vi "findMark&&ServiceItems.vi"(0 "priceListData":string[][](array[string]), 7 "Numeric":i32, 11 "error in (no error)":errorcluster) -> (8 "found?":bool, 15 "error IO":errorcluster)   [LabVIEW 2012]
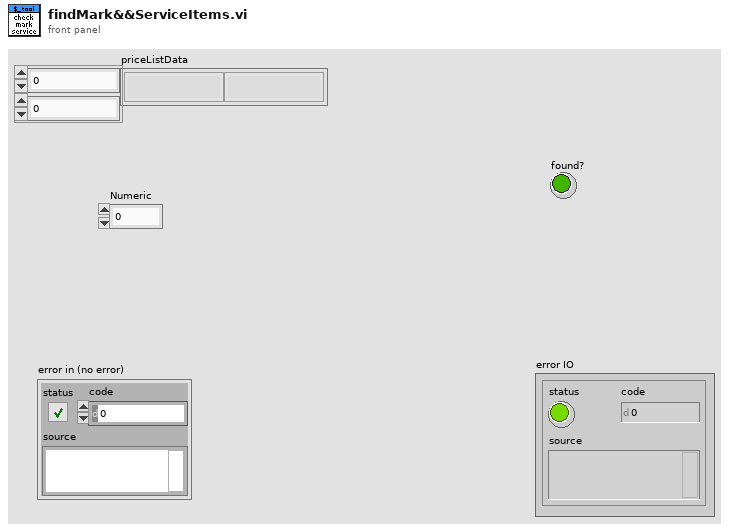
[diagram p1: front panel]
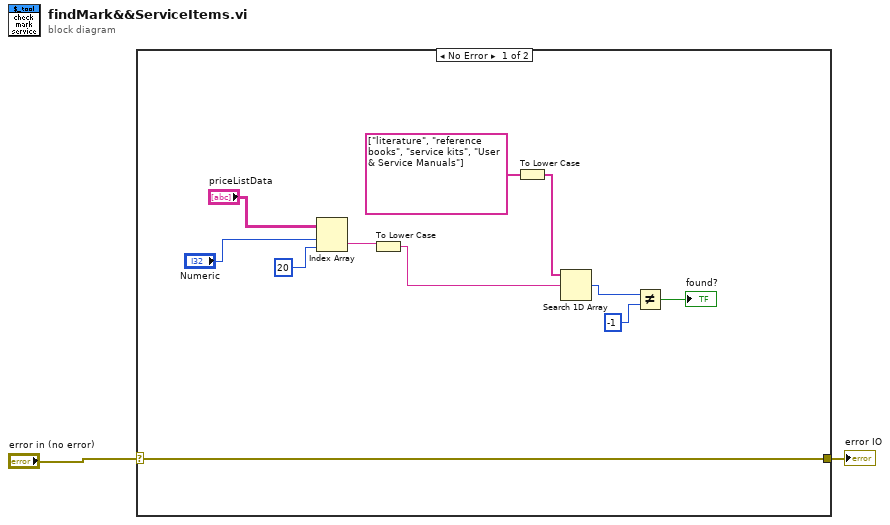
[diagram p0: block diagram]
diagram:
  n1 = case shown="No Error" "error in (no error)" {
    selector: "error in (no error)" -> [w13 w14]
    tunnel: [w13 w14] -> w1
    frame No Error {
      n2 = Index Array(array="priceListData", index (row)="Numeric", index (col)=20 ("disabled index (col)")) -> (element=w9:string)
      n3 = To Lower Case(string=w9) -> (all lower case string=w8:string)
      n4 = To Lower Case(string=string[] ["literature", "reference books", "service kits", "User & Service Manuals"]) -> (all lower case string=w3:string[])
      n5 = Search 1D Array(1D array=w3, element=w8) -> (index of element=w7:i32)  [unwired: 1 in]
      n6 = Not Equal?(x=w7, y=-1 ("index of element")) -> (x != y?=→"found?":bool)
    }
    frame Error {
    }
  }
  "error IO" <- w1
